vi "Read Lossless.vi"(0 "Depth (Unlimited)":i32=-1, 2 "Connection":refnum<class "Connection.lvclass">, 3 "Timeout mS (-1)":i32=-1, 4 "Release?":bool) -> (5 "Timed Out?":bool, 6 "Element":T1, 7 "Closed?":bool)   [LabVIEW 2020, in "Connection.lvclass"]
uses:
  Connection.lvclass
  Element.ctl
  Connection.lvclass/Connection.ctl
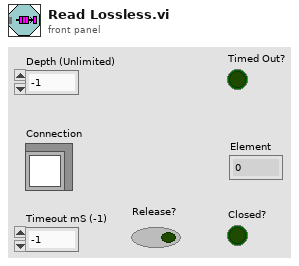
[diagram p1: front panel]
types:
  T1 = typedef "Connection.lvclass/Element.ctl" = dbl
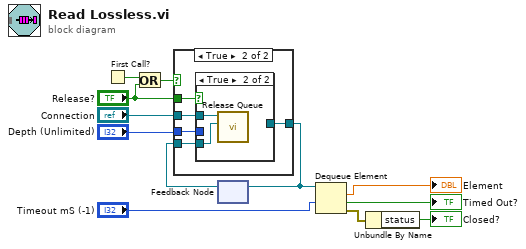
[diagram p0: block diagram]
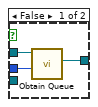
[diagram p3: hidden frame]
diagram:
  n1 = First Call?() -> (First Call?: T/F=w12:bool)
  n2 = Or(x=w12, y="Release?") -> (x .or. y?=w11:bool)
  n3 = feedback #1() -> (w7:refnum<queue>)  [unwired: 1 in]
  n4 = case shown="True" w11 {
    tunnel: "Release?" -> [_ w18]
    tunnel: "Connection" -> [_ w17]
    tunnel: [w13 w16] -> w6
    tunnel: "Depth (Unlimited)" -> [_ w15]
    tunnel: w7 -> [w13 w14]
    frame False {
    }
    frame True {
      n5 = case shown="True" w18 {
        tunnel: w17 -> [w21 w23]
        tunnel: [w20 _] -> w16
        tunnel: w15 -> [w19 _]
        tunnel: w14 -> [_ w22]
        frame False {
          n6 = call "Obtain Queue.vi"("Depth"=w19, "Connection in"=w21) -> ("Queue"=w20:refnum<queue>)  [unwired: 7 in, 2 out]
        }
        frame True {
          n7 = call "Release Queue.vi"("Queue"=w22, "Connection in"=w23) -> ()  [unwired: 8 in, 2 out]
        }
      }
    }
  }
  n8 = feedback-in #1(w6) -> ()
  n9 = Dequeue Element(queue=w6, timeout in ms (-1)="Timeout mS (-1)") -> (element=→"Element":T1, timed out?=→"Timed Out?":bool, error out=w2:errorcluster)  [unwired: 1 in, 1 out]
  n10 = Unbundle By Name(w2) -> ("status"=→"Closed?":bool)
